vi "New.vi"(7 "CreateMethod(Create or look up existing)":T1(ring), 8 "error in (no error)":errorcluster, 10 "Object name":string, 11 "reference in":refnum<class "Test_Sim.lvclass">) -> (0 "error out":errorcluster, 3 "reference out":refnum<class "Test_Sim.lvclass">, 5 "NewObjectCreated":bool)   [LabVIEW 2020, in "Test_Sim.lvlib" / "Test_Sim.lvclass"]
uses:
  Test_Sim.lvclass
  ObjectAttributes.ctl
  Config.ctl
  Test_Sim.lvclass/Test_Sim.ctl
  Components/Test_Base.lvlibp/Test_Base.lvclass
panel:
  in  "DVRRef(Hidden)":refnum<data-value>
  in  "Data":T2
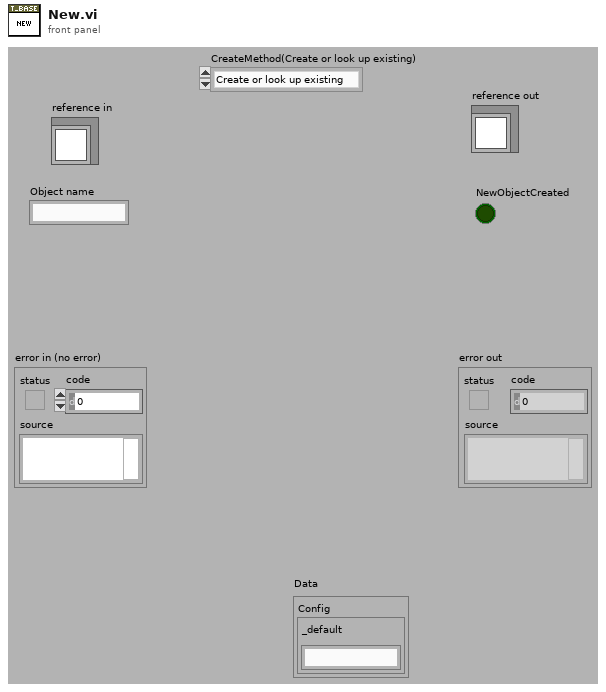
[diagram p1: front panel]
types:
  T1 = enum16{"Create or look up existing", "Look up existing"}
  T2 = typedef "Test_Sim.lvlib/Test_Sim.lvclass/ObjectAttributes.ctl" = cluster{"Config":T3}
  T3 = typedef "Test_Sim.lvlib/Test_Sim.lvclass/Config.ctl" = cluster{"_default":string}
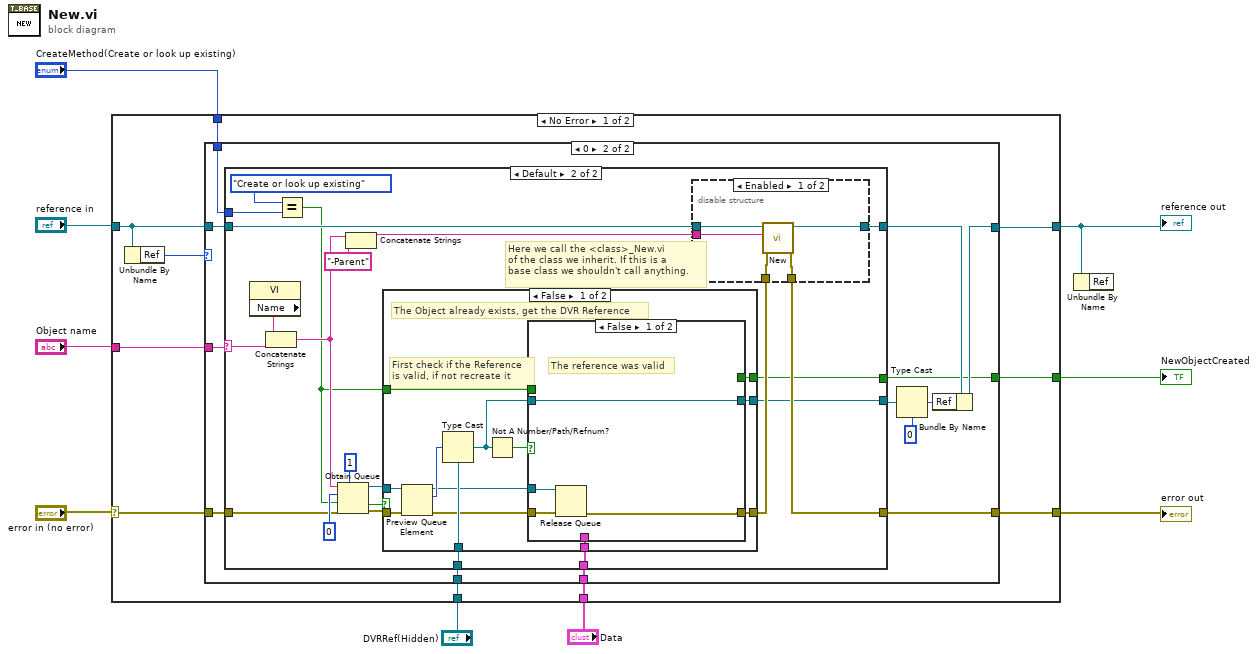
[diagram p0: block diagram]
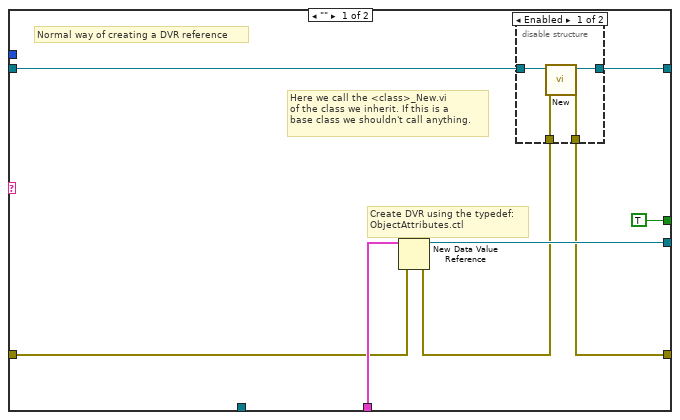
[diagram p3: hidden frame]
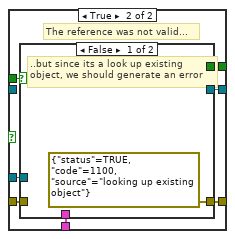
[diagram p5: hidden frame]
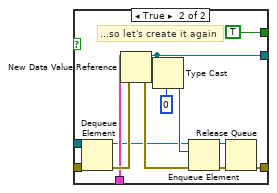
[diagram p6: hidden frame]
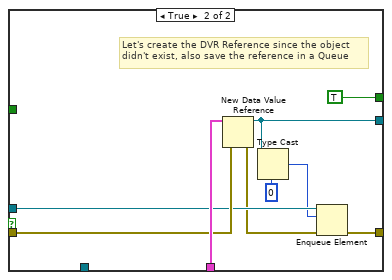
[diagram p7: hidden frame]
diagram:
  n1 = case shown="No Error" "error in (no error)" {
    selector: "error in (no error)" -> [w19 w126]
    tunnel: [w16 w126] -> w5
    tunnel: "CreateMethod(Create or look up existing)" -> [w17 _]
    tunnel: "Object name" -> [w18 _]
    tunnel: "Data" -> [w15 _]
    tunnel: "DVRRef(Hidden)" -> [w14 _]
    tunnel: "reference in" -> [w13 w125]
    tunnel: [w12 w125] -> w2
    tunnel: [w11 _] -> w3
    frame No Error {
      n2 = Unbundle By Name(w13) -> ("Ref"=w10:u32)
      n3 = case shown="0" w10 {
        tunnel: w19 -> [w21 w25]
        tunnel: w18 -> [_ w34]
        tunnel: w17 -> [_ w33]
        tunnel: [w21 w32] -> w16
        tunnel: w15 -> [_ w31]
        tunnel: w13 -> [w20 w29]
        tunnel: [w20 w30] -> w12
        tunnel: w14 -> [_ w27]
        tunnel: [_ w26] -> w11
        frame Default {
          # "The DVR reference has already been created, from this child class's <Child>_New.vi"
        }
        frame 0 {
          n4 = case shown="Default" w34 {
            selector: w34 -> [_ w62]
            tunnel: [w37 w59] -> w32
            tunnel: w33 -> [_ w69]
            tunnel: w31 -> [w42 w53]
            tunnel: [w40 w51] -> w23
            tunnel: w29 -> [w35 w68]
            tunnel: [w39 w67] -> w28
            tunnel: w27 -> [_ w54]
            tunnel: [TRUE ("created new?") w50] -> w26
            tunnel: w25 -> [w41 w60]
            frame "" {
              # "Create DVR using the typedef:\nObjectAttributes.ctl"
              # "Here we call the <class>_New.vi\nof the class we inherit. If this is a\nbase class we shouldn't call anything."
              # "Normal way of creating a DVR reference"
              n5 = New Data Value Reference(data value=w42, error in=w41) -> (data value reference=w40:refnum<data-value>, error out=w38:errorcluster)
              n6 = disable-structure shown="Enabled" {
                disable-tunnel: w35 -> [w44 w48]
                disable-tunnel: [w43 w48] -> w39
                disable-tunnel: w38 -> [w46 w47]
                disable-tunnel: [w45 w47] -> w37
                frame Enabled {
                  n7 = call-parent "New.vi"("error in (no error)"=w46, "reference in"=w44) -> ("error out"=w45:errorcluster, "reference out"=w43:refnum<class "Test_Sim.lvclass">)  [unwired: 7 in, 1 out]
                }
                frame Disabled {
                }
              }
            }
            frame Default {
              # "Here we call the <class>_New.vi\nof the class we inherit. If this is a\nbase class we shouldn't call anything."
              n8 = property class="VI"() -> ("Name"=w63:string)  [unwired: 2 in, 2 out]
              n9 = Concatenate Strings(w63, w62) -> (w61:string)
              n10 = Equal?(x=T1."Create or look up existing", y=w69) -> (x = y?=w55:bool)
              n11 = Obtain Queue(max queue size (-1, unlimited)=1, name (unnamed)=w61, element data type=u32 0 ("DataRef"), create if not found? (T)=w55, error in (no error)=w60) -> (queue out=w56:refnum<queue>, created new?=w57:bool, error out=w58:errorcluster)
              n12 = Concatenate Strings(w61, "-Parent" ("string")) -> (w64:string)
              n13 = case shown="False" w57 {
                tunnel: w58 -> [w82 w116]
                tunnel: w53 -> [w73 w117]
                tunnel: w56 -> [w83 w115]
                tunnel: [w77 w112] -> w52
                tunnel: [w75 w111] -> w51
                tunnel: w54 -> [w80 _]
                tunnel: [w72 TRUE] -> w50
                tunnel: w55 -> [w71 _]
                frame False {
                  # "First check if the Reference\nis valid, if not recreate it"
                  # "The Object already exists, get the DVR Reference"
                  n14 = Preview Queue Element(queue=w83, error in (no error)=w82) -> (queue out=w74:refnum<queue>, element=w81:u32, error out=w79:errorcluster)  [unwired: 1 in, 1 out]
                  n15 = Type Cast(type=w80, x=w81) -> (*(type *) &x=w76:refnum<data-value>)
                  n16 = Not A Number/Path/Refnum?(number/path/refnum=w76) -> (NaN/Path/Refnum?=w78:bool)
                  n17 = case shown="False" w78 {
                    tunnel: w79 -> [w85 w93]
                    tunnel: [w84 w90] -> w77
                    tunnel: w76 -> [w87 _]
                    tunnel: [w87 w91] -> w75
                    tunnel: w74 -> [w86 w94]
                    tunnel: w73 -> [_ w92]
                    tunnel: [_ w89] -> w72
                    tunnel: w71 -> [_ w88]
                    frame False {
                      # "The reference was valid"
                      n18 = Release Queue(queue=w86, error in (no error)=w85) -> (error out=w84:errorcluster)  [unwired: 1 in, 2 out]
                    }
                    frame True {
                      # "The reference was not valid..."
                      n19 = case shown="False" w88 {
                        tunnel: w94 -> [_ w108]
                        tunnel: w93 -> [_ w107]
                        tunnel: w92 -> [_ w103]
                        tunnel: [_ w100] -> w91
                        tunnel: [errorcluster {"status"=TRUE, "code"=1100, "source"="looking up existing object"} ("error out") w96] -> w90
                        tunnel: [_ TRUE] -> w89
                        frame False {
                          # "..but since its a look up existing\nobject, we should generate an error"
                        }
                        frame True {
                          # "...so let's create it again"
                          n20 = Dequeue Element(queue=w108, error in (no error)=w107) -> (queue out=w101:refnum<queue>, error out=w104:errorcluster)  [unwired: 1 in, 2 out]
                          n21 = New Data Value Reference(data value=w103, error in=w104) -> (data value reference=w100:refnum<data-value>, error out=w102:errorcluster)
                          n22 = Type Cast(type=u32 0 ("ObjectQueue"), x=w100) -> (*(type *) &x=w105:u32)
                          n23 = Enqueue Element(queue=w101, element=w105, error in (no error)=w102) -> (queue out=w97:refnum<queue>, error out=w98:errorcluster)  [unwired: 1 in, 1 out]
                          n24 = Release Queue(queue=w97, error in (no error)=w98) -> (error out=w96:errorcluster)  [unwired: 1 in, 2 out]
                        }
                      }
                    }
                  }
                }
                frame True {
                  # "Let's create the DVR Reference since the object\ndidn't exist, also save the reference in a Queue"
                  n25 = New Data Value Reference(data value=w117, error in=w116) -> (data value reference=w111:refnum<data-value>, error out=w113:errorcluster)
                  n26 = Type Cast(type=u32 0 ("ObjectQueue"), x=w111) -> (*(type *) &x=w110:u32)
                  n27 = Enqueue Element(queue=w115, element=w110, error in (no error)=w113) -> (error out=w112:errorcluster)  [unwired: 1 in, 2 out]
                }
              }
              n28 = disable-structure shown="Enabled" {
                disable-tunnel: w68 -> [w120 w124]
                disable-tunnel: [w118 w124] -> w67
                disable-tunnel: w64 -> [w119 _]
                disable-tunnel: w52 -> [w122 w123]
                disable-tunnel: [w121 w123] -> w59
                frame Enabled {
                  n29 = call-parent "New.vi"("error in (no error)"=w122, "Object name"=w119, "reference in"=w120) -> ("error out"=w121:errorcluster, "reference out"=w118:refnum<class "Test_Sim.lvclass">)  [unwired: 6 in, 1 out]
                }
                frame Disabled {
                }
              }
            }
          }
          n30 = Type Cast(type=u32 0 ("DataRef"), x=w23) -> (*(type *) &x=w22:u32)
          n31 = Bundle By Name(cluster=w28, "Ref"=w22) -> (w30:refnum<class "Test_Sim.lvclass">)
        }
      }
    }
    frame Error {
    }
  }
  "error out" <- w5
  "reference out" <- w2
  "NewObjectCreated" <- w3
  n32 = Unbundle By Name(w2) -> ()  [unwired: 1 out]
